vi "GetTask.vi"(8 "error in (no error)":errorcluster, 10 "task":dbl, 11 "Database in":refnum<class "Database.lvclass">) -> (0 "error out":errorcluster, 2 "task params":T1(array[cluster]), 3 "Database out":refnum<class "Database.lvclass">)   [LabVIEW 2014, in "Database.lvclass"]
uses:
  Database.lvclass
  Database.lvclass/Database.ctl
  <vilib>/addons/database/_DB Variant To Data/Database Variant To Data.xnode
  <vilib>/addons/database/NI_Database_API.lvlib
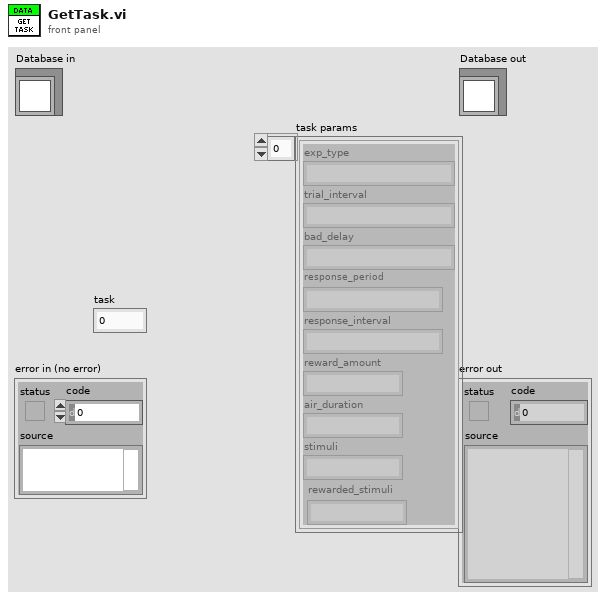
[diagram p1: front panel]
types:
  T1 = cluster{"exp_type":string, "trial_interval":string, "bad_delay":string, "response_period":string, "response_interval":string, "reward_amount":string, "air_duration":string, "stimuli":string, "rewarded_stimuli":string}[]
  T2 = typedef "NI_Database_API.lvlib/Conn ObjectReference.ctl" = refnum<k1>
  T3 = cluster{"data[0]":string, "data[1]":string, "data[2]":string, "data[3]":string, "data[4]":string, "data[5]":string, "data[6]":string, "data[7]":string, "data[8]":string}
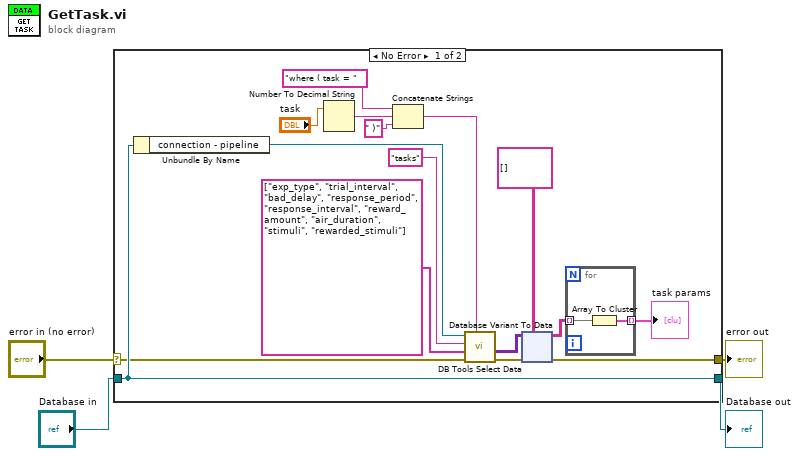
[diagram p0: block diagram]
diagram:
  n1 = case shown="No Error" "error in (no error)" {
    selector: "error in (no error)" -> [w12 w68]
    tunnel: [w10 w68] -> w3
    tunnel: [w14 w67] -> w1
    tunnel: "Database in" -> [w14 w67]
    frame No Error {
      n2 = Unbundle By Name(w14) -> ("connection - pipeline"=w13:T2)
      n3 = Number To Decimal String(number="task") -> (decimal integer string=w9:string)  [unwired: 1 in]
      n4 = Concatenate Strings("where ( task = ", w9, " )") -> (w7:string)
      n5 = call <vilib>:"DB Tools Select Data.vi"("condition"=w7, "error in (no error)"=w12, "columns"=string[] ["exp_type", "trial_interval", "bad_delay", "response_period", "response_interval", "reward_amount", "air_duration", "stimuli", "rewarded_stimuli"], "table"="tasks", "connection reference"=w13) -> ("error out"=w11:errorcluster, "data"=w16:variant[][])  [unwired: 1 in, 1 out]
      n6 = xnode "Database Variant To Data"("database variant"=w16, "error in (no error)"=w11, "type"=string[][] []) -> ("data"=w18:string[][], "error out"=w10:errorcluster)
      n7 = for {
        tunnel: w18 -> [w22] mode=indexing
        tunnel: [w21] -> w6 mode=indexing
        n8 = Array To Cluster(array=w22) -> (cluster=w21:T3)
      }
      "task params" <- w6
    }
    frame Error {
    }
  }
  "error out" <- w3
  "Database out" <- w1
